vi "Conf_select.vi"(1 "Config":string="DTU_EOL") -> (0 "index of element":i32)   [LabVIEW 2024, in "Test_2.lvlib"]
uses:
  Test_2.lvlib
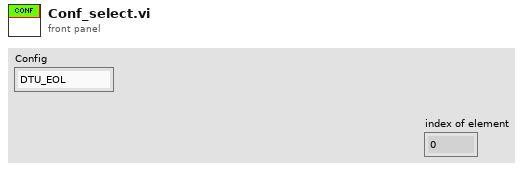
[diagram p1: front panel]
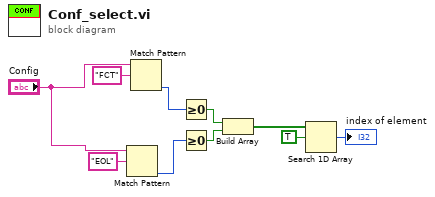
[diagram p0: block diagram]
diagram:
  n1 = Match Pattern(string="Config", regular expression="EOL") -> (offset past match=w7:i32)  [unwired: 1 in, 3 out]
  n2 = Match Pattern(string="Config", regular expression="FCT") -> (offset past match=w8:i32)  [unwired: 1 in, 3 out]
  n3 = Greater Or Equal To 0?(x=w8) -> (x >= 0?=w5:bool)
  n4 = Greater Or Equal To 0?(x=w7) -> (x >= 0?=w6:bool)
  n5 = Build Array(w5, w6) -> (w4:bool[])
  n6 = Search 1D Array(1D array=w4, element=TRUE) -> (index of element=→"index of element":i32)  [unwired: 1 in]
